vi "Logging Cases.vi"(0 "Logging queue":refnum<queue>, 1 "Channel info":T1, 2 "Enable ref saving during functional acq.":bool, 3 "Number of files closed in":u32, 5 "Logging queue element in":T6={"Imaging Protocol"=enum."Live Imaging", "Number of Trials"=0, "Frame Size"=512, "# Averaged frames"=0, "Dwell time (us)"=0.0, "Index of Z-plane"=0, "Timelapse?"=FALSE, "Logging process is active"=FALSE, "Speed logging enabled"=FALSE, "tdms file ref"=refnum, "path"=path "", "Trial Number"=0, "Expected # points acquired"=FALSE, "Manually stopped"=FALSE, "Last trial"=FALSE, "Ch0 data"=[], "Ch1 data"=[], "Ref Data"=[], "Ref Frame Time"=[], "Image Time"=[], "Continuous Time"=[], "Ref X Length"=0, "Ref Y Length"=0, "# Ref Averaged frames"=0, "Ref Dwell time (us)"=0.0, "Points acquired"={"Ch0 last trial"=0, "Ch1 last trial"=0, "All trials"=0}, "HW Timings File"=refnum} {"Ref Dwell time (us)" format="%#.6g"; "Frame Size" items=["100X100"=100, "128X128"=128, "200X200"=200, "256X256"=256, "512X512"=512, "1024x1024"=1024, "2048x2048"=2048]; "Dwell time (us)" format="%#.6g"}, 7 "UI queue":refnum<queue>, 9 "Data-gen queue":T5, 11 "error in":errorcluster, 12 "Live graph data queue in":T2, 14 "Image array":T3) -> (6 "Number of TDMS files closed":u32, 15 "error out":errorcluster)   [LabVIEW 2017]
uses:
  Typedefs/Logging queue element.ctl
  Typedefs/Imaging Protocols enum.ctl
  Typedefs/Frame Size.ctl
  Typedefs/Acquired points count.ctl
  Typedefs/ROI File Generator Queue Ref.ctl
  User Interface/Queue/Live graphs queue/Typedefs/Live imaging queue element.ctl
  <vilib>/vision/Image Controls.llb/IMAQ Image.ctl
  User Interface/Typedefs/Live graph data queue ref.ctl
  User Interface/Queue/Message Queue/Typedefs/Message Cluster.ctl
panel:
  out "Number of points in completed Ref frame":i32
  out "Number of points in completed standard frame":i32
  out "Peak # points received":dbl
  out "# points received":i32
  # "<-- For debugging only"
  # "<-- For debugging only"
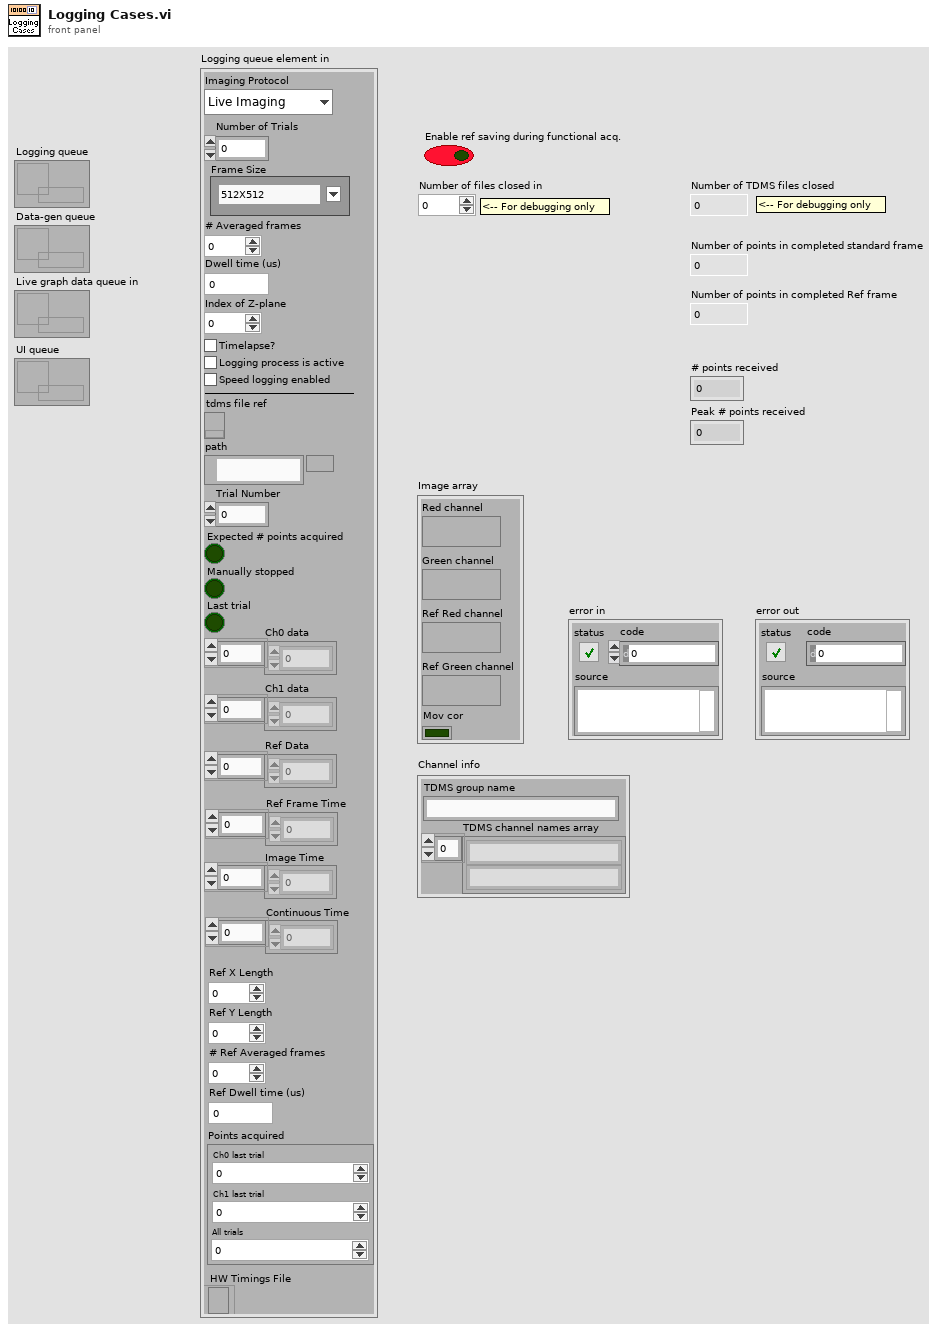
[diagram p1: front panel]
types:
  T1 = cluster{"TDMS group name":string, "TDMS channel names array":string[]}
  T2 = typedef "Live graph data queue ref.ctl" = refnum<queue>
  T3 = typedef "Live imaging queue element.ctl" = cluster{"Red channel":T4, "Green channel":T4, "Ref Red channel":T4, "Ref Green channel":T4, "Mov cor":bool}
  T4 = typedef "IMAQ Image.ctl" = refnum<image>
  T5 = typedef "ROI File Generator Queue Ref.ctl" = refnum<queue>
  T6 = typedef "Logging queue element.ctl" = cluster{"Imaging Protocol":T7, "Number of Trials":u16, "Frame Size":T8, "# Averaged frames":u16, "Dwell time (us)":dbl, "Index of Z-plane":i32, "Timelapse?":bool, "Logging process is active":bool, "Speed logging enabled":bool, "tdms file ref":refnum<k34>, "path":path, "Trial Number":i32, "Expected # points acquired":bool, "Manually stopped":bool, "Last trial":bool, "Ch0 data":u32[], "Ch1 data":u32[], "Ref Data":u32[], "Ref Frame Time":u64[], "Image Time":u64[], "Continuous Time":u64[], "Ref X Length":u16, "Ref Y Length":u16, "# Ref Averaged frames":u16, "Ref Dwell time (us)":dbl, "Points acquired":T9, "HW Timings File":refnum<file>}
  T7 = typedef "Imaging Protocols enum.ctl" = enum16{"AOL Z-Stack", "Motor Z Stack", "Functional Acquisition", "Single Plane Acquisition", "Volume Acquisition", "Live Imaging", "Live Plane Imaging", "Live Volume Imaging"}
  T8 = typedef "Frame Size.ctl" = u16
  T9 = typedef "Acquired points count.ctl" = cluster{"Ch0 last trial":u64, "Ch1 last trial":u64, "All trials":u64}
  T10 = typedef "Frame data dual cluster.ctl" = cluster{"Red channel frame":dbl[], "Green channel frame":dbl[], "Red channel Ref":dbl[], "Green channel Ref":dbl[]}
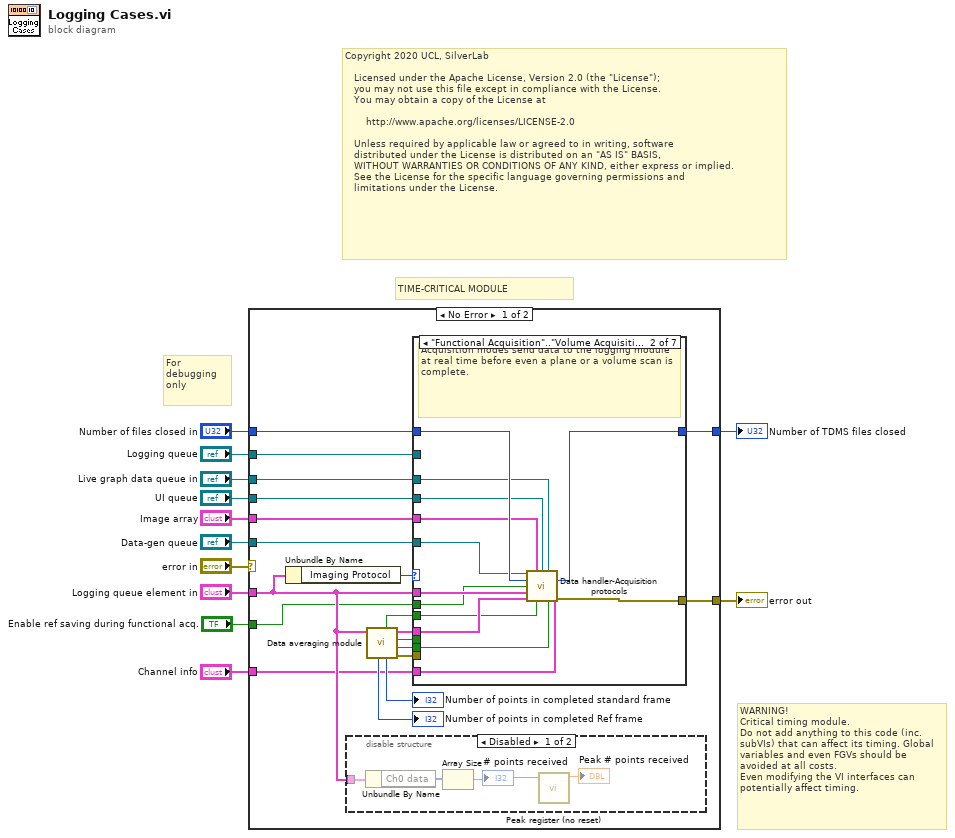
[diagram p0: block diagram]
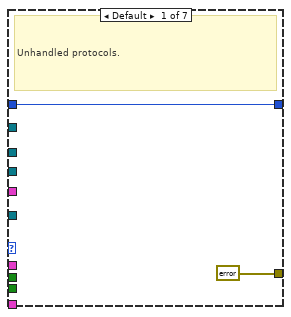
[diagram p2: hidden frame]
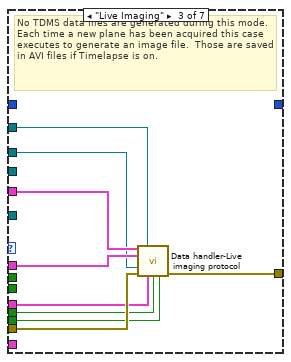
[diagram p3: hidden frame]
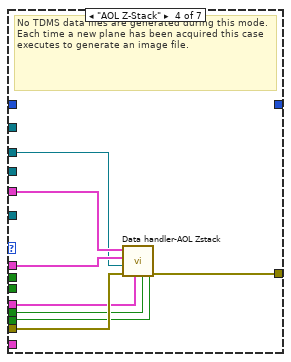
[diagram p4: hidden frame]
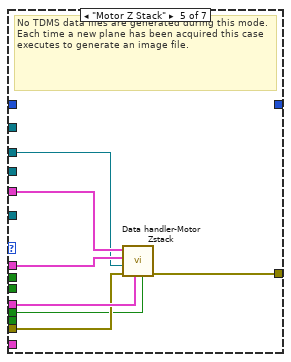
[diagram p5: hidden frame]
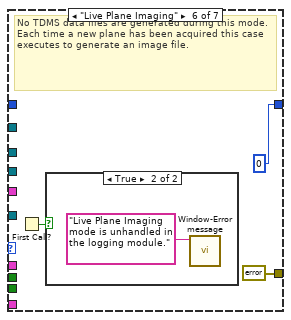
[diagram p6: hidden frame]
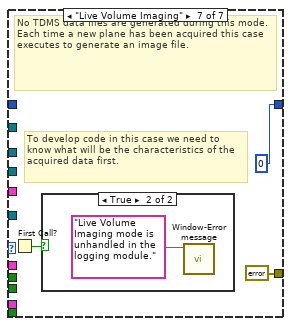
[diagram p8: hidden frame]
diagram:
  # "Copyright 2020 UCL, SilverLab\n \n   Licensed under the Apache License, Version 2.0 (the \"License\");\n   you may not use this file except in compliance with the License.\n   You may obtain a copy of the License at\n \n       http://www.apache.org/licenses/LICENSE-2.0\n \n   Unless required by applicable law or agreed to in writing, software\n   distributed under the License is distributed on an \"AS IS\" BASIS,\n   WITHOUT WARRANTIES OR CONDITIONS OF ANY KIND, either express or implied.\n   See the License for the specific language governing permissions and\n   limitations under the License."
  # "TIME-CRITICAL MODULE"
  # "WARNING!\nCritical timing module.\nDo not add anything to this code (inc. subVIs) that can affect its timing. Global variables and even FGVs should be avoided at all costs.\nEven modifying the VI interfaces can potentially affect timing."
  # "For debugging only"
  n1 = case shown="No Error" "error in" {
    selector: "error in" -> [_ w83]
    tunnel: "Number of files closed in" -> [w31 _]
    tunnel: [w30 _] -> w11
    tunnel: "Data-gen queue" -> [w29 _]
    tunnel: [w28 w83] -> w9
    tunnel: "Logging queue element in" -> [w21 _]
    tunnel: "Image array" -> [w26 _]
    tunnel: "Live graph data queue in" -> [w25 _]
    tunnel: "Channel info" -> [w16 _]
    tunnel: "Enable ref saving during functional acq." -> [w15 _]
    tunnel: "Logging queue" -> [w14 _]
    tunnel: "UI queue" -> [w13 _]
    frame No Error {
      n2 = Unbundle By Name(w21) -> ("Imaging Protocol"=w27:T7)
      n3 = disable-structure shown="Disabled" {
        disable-tunnel: w21 -> [w79 _]
        frame Disabled {
          n4 = Unbundle By Name(w79) -> ("Ch0 data"=w80:u32[])
          n5 = Array Size(array=w80) -> (size(s)=w81:i32)
          "# points received" <- w81
          n6 = call <userlib>:"Peak register (no reset).vi"("Value in"=w81) -> ("Registered peak value"=→"Peak # points received":dbl)  [unwired: 10 in]
        }
        frame Enabled {
        }
      }
      n7 = call "Data averaging module.vi"("Logging queue element in"=w21) -> ("error out"=w24:errorcluster, "Ref Frame completed/generate image"=w20:bool, "Standard Frame completed/generate image"=w22:bool, "Single Frame Data"=w23:T10, "Number of points in completed standard frame"=→"Number of points in completed standard frame":i32, "Movement Correction"=w17:bool, "Number of points in completed Ref frame"=→"Number of points in completed Ref frame":i32)  [unwired: 4 in]
      n8 = case shown="\"Functional Acquisition\"..\"Volume Acquisition\"" w27 {
        tunnel: w31 -> [w33 w46 _ _ _ _ _]
        tunnel: [w33 w42 _ _ _ u32 0 ("Number of files closed in") u32 0 ("Number of files closed in")] -> w30
        tunnel: w29 -> [_ w45 _ _ _ _ _]
        tunnel: [errorcluster {"status"=FALSE, "code"=0, "source"=""} ("error out") w44 w53 w61 w69 errorcluster {"status"=FALSE, "code"=0, "source"=""} ("error out") errorcluster {"status"=FALSE, "code"=0, "source"=""} ("error out")] -> w28
        tunnel: w21 -> [_ w43 w54 w62 w68 _ _]
        tunnel: w26 -> [_ w40 w55 w63 w70 _ _]
        tunnel: w25 -> [_ w39 w52 w57 w64 _ _]
        tunnel: w24 -> [_ _ w51 w60 w66 _ _]
        tunnel: w23 -> [_ w41 w50 w59 w67 _ _]
        tunnel: w22 -> [_ _ w49 w58 w65 _ _]
        tunnel: w20 -> [_ w38 w48 w56 _ _ _]
        tunnel: w17 -> [_ w37 _ _ _ _ _]
        tunnel: w16 -> [_ w36 _ _ _ _ _]
        tunnel: w15 -> [_ w35 _ _ _ _ _]
        tunnel: w14 -> [_ _ w47 _ _ _ _]
        tunnel: w13 -> [_ w34 _ _ _ _ _]
        frame Default {
          # "Unhandled protocols."
        }
        frame "Functional Acquisition".."Volume Acquisition" {
          # "Acquisition modes send data to the logging module at real time before even a plane or a volume scan is complete."
          n9 = call "Data handler-Acquisition protocols.vi"("Data-gen queue"=w45, "Image array"=w40, "UI queue"=w34, "Live graph data queue in"=w39, "Channel info"=w36, "Number of files closed in in"=w46, "Enable ref saving"=w35, "Logging queue element in"=w43, "Single Frame Data"=w41, "Movement Correction"=w37, "Save Reference"=w38) -> ("Number of files closed out"=w42:u32, "error out"=w44:errorcluster)  [unwired: 3 in]
        }
        frame "Live Imaging" {
          # "No TDMS data files are generated during this mode.  Each time a new plane has been acquired this case executes to generate an image file.  Those are saved in AVI files if Timelapse is on."
          n10 = call "Data handler-Live imaging protocol.vi"("Image array"=w55, "Logging queue"=w47, "Logging queue element in"=w54, "Live graph data queue in"=w52, "error in (no error)"=w51, "Single Frame Data"=w50, "Frame completed/generate image"=w49, "RefFrame completed/generate image"=w48) -> ("error out"=w53:errorcluster)  [unwired: 7 in]
        }
        frame "AOL Z-Stack" {
          # "No TDMS data files are generated during this mode. Each time a new plane has been acquired this case executes to generate an image file."
          n11 = call "Data handler-AOL Zstack.vi"("Save image"=w58, "Save Ref image"=w56, "Single Frame Data"=w59, "error in (no error)"=w60, "Live graph data queue in"=w57, "Logging queue element in"=w62, "Image array"=w63) -> ("error out"=w61:errorcluster)  [unwired: 4 in]
        }
        frame "Motor Z Stack" {
          # "No TDMS data files are generated during this mode. Each time a new plane has been acquired this case executes to generate an image file."
          n12 = call "Data handler-Motor Zstack.vi"("Save image"=w65, "Single Frame Data"=w67, "error in (no error)"=w66, "Live graph data queue in"=w64, "Logging queue element in"=w68, "Image array"=w70) -> ("error out"=w69:errorcluster)  [unwired: 5 in]
        }
        frame "Live Plane Imaging" {
          # "No TDMS data files are generated during this mode. Each time a new plane has been acquired this case executes to generate an image file."
          n13 = First Call?() -> (First Call?: T/F=w71:bool)
          n14 = case shown="True" w71 {
            frame False {
            }
            frame True {
              n15 = call "Window-Error message.vi"("Message"="Live Plane Imaging mode is unhandled in the logging module." ("message")) -> ()  [unwired: 10 in, 1 out]
            }
          }
        }
        frame "Live Volume Imaging" {
          # "To develop code in this case we need to know what will be the characteristics of the acquired data first."
          # "No TDMS data files are generated during this mode. Each time a new plane has been acquired this case executes to generate an image file."
          n16 = First Call?() -> (First Call?: T/F=w75:bool)
          n17 = case shown="True" w75 {
            frame False {
            }
            frame True {
              n18 = call "Window-Error message.vi"("Message"="Live Volume Imaging mode is unhandled in the logging module." ("message")) -> ()  [unwired: 10 in, 1 out]
            }
          }
        }
      }
    }
    frame Error {
    }
  }
  "Number of TDMS files closed" <- w11
  "error out" <- w9
